vi "Tx Disable channel logic 2ch.vi"(5 "num channels":u32, 6 "ready for output":bool, 9 "input valid":bool, 10 "data in":u32[](array[numeric])=[0, 0, 0, 0], 11 "enabled channels":u32) -> (0 "enable new data":bool, 1 "output valid":bool, 2 "data out":u32[](array[numeric]))   [LabVIEW 2025, in "niUSRP Stream Control (DMA) v1 FPGA.lvclass"]
uses:
  niUSRP Stream Control (DMA) v1 FPGA.lvclass
  niUSRP Stream Control (DMA) v1 FPGA.lvclass/niUSRP Stream Control (DMA) v1 FPGA.ctl
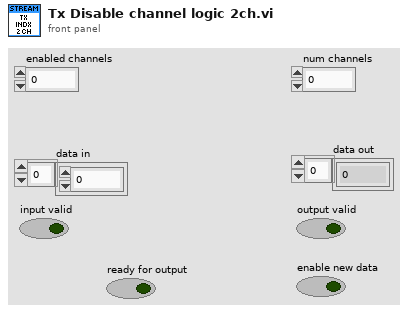
[diagram p1: front panel]
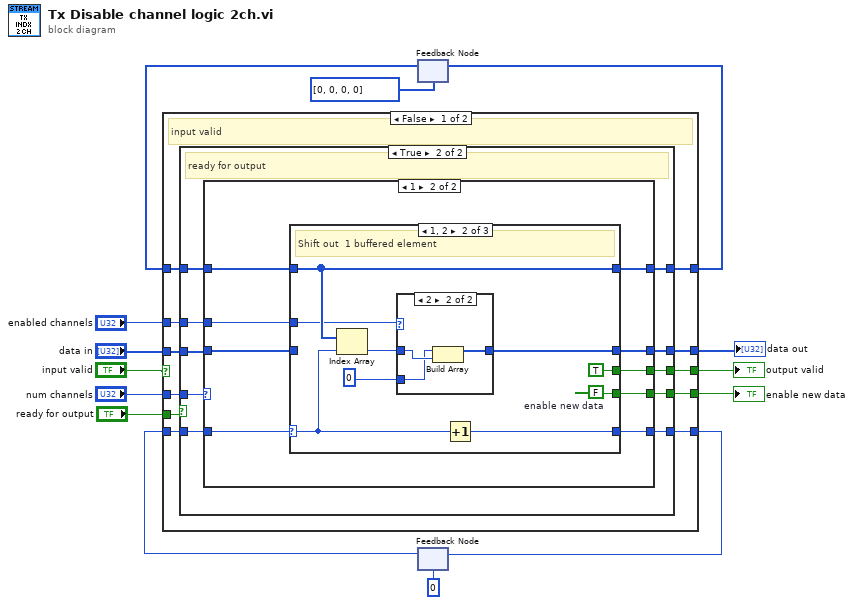
[diagram p0: block diagram]
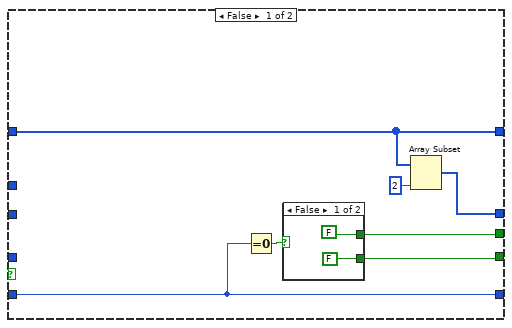
[diagram p2: hidden frame]
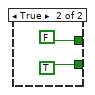
[diagram p3: hidden frame]
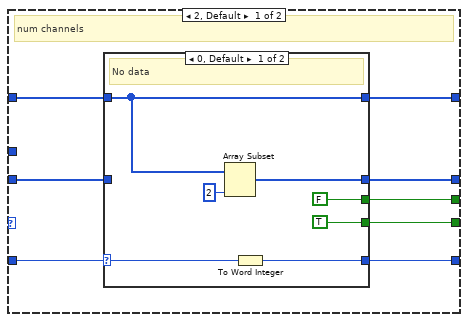
[diagram p4: hidden frame]
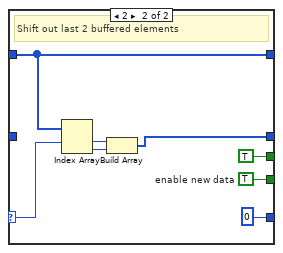
[diagram p5: hidden frame]
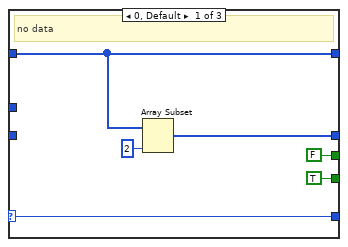
[diagram p6: hidden frame]
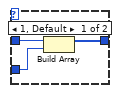
[diagram p7: hidden frame]
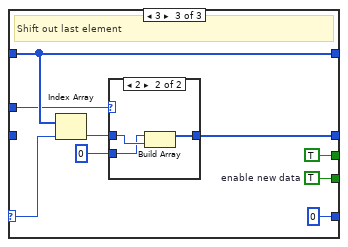
[diagram p8: hidden frame]
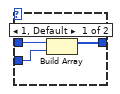
[diagram p9: hidden frame]
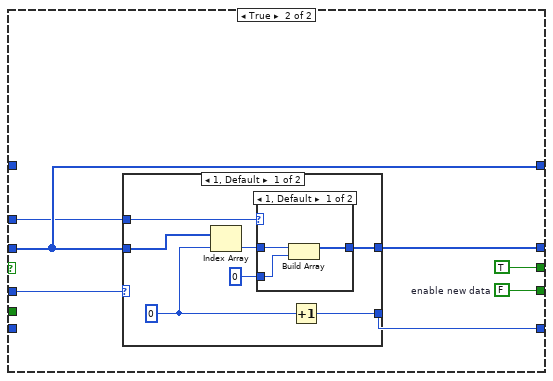
[diagram p10: hidden frame]
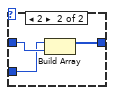
[diagram p11: hidden frame]
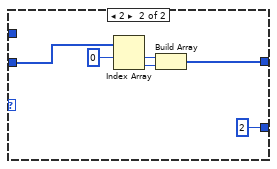
[diagram p12: hidden frame]
diagram:
  n1 = feedback #1(u32[] [0, 0, 0, 0]) -> (w6:u32[])
  n2 = feedback #2(i16 0) -> (w2:i16)
  n3 = case shown="False" "input valid" {
    tunnel: [w25 w119] -> w14
    tunnel: [w24 TRUE] -> w13
    tunnel: [w23 w121] -> w12
    tunnel: "data in" -> [w22 w116]
    tunnel: "enabled channels" -> [w21 w115]
    tunnel: "num channels" -> [w20 w117]
    tunnel: w6 -> [w19 _]
    tunnel: [w17 w116] -> w5
    tunnel: [w16 w118] -> w3
    tunnel: w2 -> [w18 _]
    tunnel: "ready for output" -> [w15 _]
    frame False {
      # "input valid"
      n4 = case shown="True" w15 {
        tunnel: [w30 w46] -> w25
        tunnel: [w31 w45] -> w24
        tunnel: [w26 w44] -> w23
        tunnel: w22 -> [_ w43]
        tunnel: w21 -> [_ w42]
        tunnel: w20 -> [_ w41]
        tunnel: w19 -> [w28 w40]
        tunnel: w18 -> [w29 w39]
        tunnel: [w28 w38] -> w17
        tunnel: [w29 w37] -> w16
        frame False {
          n5 = Equal To 0?(x=w29) -> (x = 0?=w32:bool)
          n6 = case shown="False" w32 {
            tunnel: [FALSE TRUE] -> w30
            tunnel: [FALSE FALSE] -> w31
            frame False {
            }
            frame True {
            }
          }
          n7 = Array Subset(array=w28, length=2) -> (w26:u32[])  [unwired: 1 in]
        }
        frame True {
          # "ready for output"
          n8 = case shown="1" w41 {
            tunnel: [w54 w76] -> w45
            tunnel: [w53 w77] -> w44
            tunnel: w43 -> [w52 w78]
            tunnel: [w51 w75] -> w46
            tunnel: w42 -> [_ w74]
            tunnel: w40 -> [w49 w71]
            tunnel: w39 -> [w50 w72]
            tunnel: [w48 w70] -> w38
            tunnel: [w47 w73] -> w37
            frame 2, Default {
              # "num channels"
              n9 = case shown="0, Default" w50 {
                selector: w50 -> [w60 w68]
                tunnel: w52 -> [_ _]
                tunnel: [w59 i16 0] -> w47
                tunnel: [w56 w63] -> w53
                tunnel: [FALSE TRUE] -> w54
                tunnel: w49 -> [w55 w67]
                tunnel: [w55 w67] -> w48
                tunnel: [TRUE w62] -> w51
                frame 0, Default {
                  # "No data"
                  n10 = Array Subset(array=w55, length=2) -> (w56:u32[])  [unwired: 1 in]
                  n11 = To Word Integer(number=w60) -> (16bit integer=w59:i16)
                }
                frame 2 {
                  w62 = TRUE  # enable new data
                  # "Shift out last 2 buffered elements"
                  n12 = Index Array(array=w67, index #1=w68) -> (element #1=w65:u32, element #2=w64:u32)  [unwired: 1 in]
                  n13 = Build Array(w65, w64) -> (w63:u32[])
                }
              }
            }
            frame 1 {
              n14 = case shown="1, 2" w72 {
                selector: w72 -> [w83 w90 w104]
                tunnel: w78 -> [_ _ _]
                tunnel: [w83 w93 i16 0] -> w73
                tunnel: [w79 w92 w101] -> w77
                tunnel: [FALSE TRUE TRUE] -> w76
                tunnel: w71 -> [w81 w89 w105]
                tunnel: [w81 w89 w105] -> w70
                tunnel: [TRUE w88 w106] -> w75
                tunnel: w74 -> [_ w86 w103]
                frame 0, Default {
                  # "no data"
                  n15 = Array Subset(array=w81, length=2) -> (w79:u32[])  [unwired: 1 in]
                }
                frame 1, 2 {
                  w88 = FALSE  # enable new data
                  # "Shift out  1 buffered element"
                  n16 = Index Array(array=w89, index=w90) -> (element=w87:u32)
                  n17 = case shown="2" w86 {
                    tunnel: [w96 w99] -> w92
                    tunnel: w87 -> [w95 w98]
                    tunnel: u32 0 -> [w94 w97]
                    frame 1, Default {
                      n18 = Build Array(w95, w94) -> (w96:u32[])
                    }
                    frame 2 {
                      n19 = Build Array(w97, w98) -> (w99:u32[])
                    }
                  }
                  n20 = Increment(x=w90) -> (x+1=w93:i16)
                }
                frame 3 {
                  w106 = TRUE  # enable new data
                  # "Shift out last element"
                  n21 = Index Array(array=w105, index=w104) -> (element=w102:u32)
                  n22 = case shown="2" w103 {
                    tunnel: [w111 w114] -> w101
                    tunnel: w102 -> [w110 w113]
                    tunnel: u32 0 -> [w109 w112]
                    frame 1, Default {
                      n23 = Build Array(w110, w109) -> (w111:u32[])
                    }
                    frame 2 {
                      n24 = Build Array(w112, w113) -> (w114:u32[])
                    }
                  }
                }
              }
            }
          }
        }
      }
    }
    frame True {
      w119 = FALSE  # enable new data
      n25 = case shown="1, Default" w117 {
        tunnel: [w123 w137] -> w121
        tunnel: w116 -> [w127 w136]
        tunnel: [w126 i16 2 ("length")] -> w118
        tunnel: w115 -> [w122 _]
        frame 1, Default {
          w128 = i16 0
          n26 = Index Array(array=w127, index=w128) -> (element=w125:u32)
          n27 = case shown="1, Default" w122 {
            tunnel: [w131 w134] -> w123
            tunnel: w125 -> [w130 w133]
            tunnel: u32 0 -> [w129 w132]
            frame 1, Default {
              n28 = Build Array(w130, w129) -> (w131:u32[])
            }
            frame 2 {
              n29 = Build Array(w132, w133) -> (w134:u32[])
            }
          }
          n30 = Increment(x=w128) -> (x+1=w126:i16)
        }
        frame 2 {
          n31 = Index Array(array=w136, index #1=0) -> (element #1=w139:u32, element #2=w138:u32)  [unwired: 1 in]
          n32 = Build Array(w139, w138) -> (w137:u32[])
        }
      }
    }
  }
  "enable new data" <- w14
  "output valid" <- w13
  "data out" <- w12
  n33 = feedback-in #1(w5) -> ()
  n34 = feedback-in #2(w3) -> ()
